vi "CAL-Interp.vi"(0 "Frequency (Hz)":dbl[](array[numeric]), 5 "Magnitude (dB)":dbl[](array[numeric]), 7 "Phase (degrees)":dbl[](array[numeric]), 9 "df (Hz)":dbl) -> (4 "Interp Freq (Hz)":dbl[](array[numeric]), 6 "Interp Magnitude (dB)":dbl[](array[numeric]), 8 "Interp Phase (degrees)":dbl[](array[numeric]), 15 "Interp z":cdb[](array[numeric]))   [LabVIEW 2020]
uses:
  epl-vi-lib/Utility VIs/Math VIs/dB to Linear (1D).vi
  epl-vi-lib/Utility VIs/Math VIs/LinSpace (start-stop-step).vi
  epl-vi-lib/Utility VIs/Math VIs/Linear to dB (array).vi
  <vilib>/gmath/NI_Gmath.lvlib
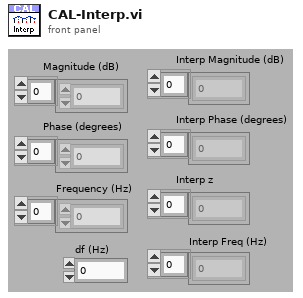
[diagram p1: front panel]
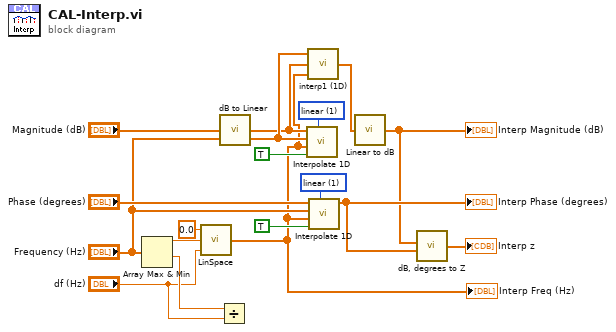
[diagram p0: block diagram]
diagram:
  w13 = 1 items=["nearest", "linear", "spline", "cubic Hermite", "Lagrange"] ("method")
  w17 = 1 items=["nearest", "linear", "spline", "cubic Hermite", "Lagrange"] ("method")
  n1 = Array Max & Min(array="Frequency (Hz)") -> (max value=w15:dbl, min value=w6:dbl)  [unwired: 2 out]
  n2 = call-poly "LinSpace.vi"("Step"="df (Hz)", "Stop"=w15, "Start"=0.0) -> ("Array"=w2:dbl[])  [unwired: 1 in, 1 out]
  "Interp Freq (Hz)" <- w2
  n3 = Divide(x=w6, y="df (Hz)") -> ()  [unwired: 1 out]
  n4 = call-poly "dB to Linear.vi"("dB"="Magnitude (dB)") -> ("linear"=w3:dbl[])
  n5 = call <vilib>:"Interpolate 1D.vi"("method"=w17, "X is monotonic"=TRUE, "xi"=w2, "X"="Frequency (Hz)", "Y"=w3) -> ()  [unwired: 4 in, 3 out]
  n6 = call "interp1 (1D).vi"("X"="Frequency (Hz)", "Y"=w3, "U"=w2) -> ("V"=w1:dbl[])  [unwired: 2 in]
  n7 = call <vilib>:"Interpolate 1D.vi"("method"=w13, "X is monotonic"=TRUE, "xi"=w2, "X"="Frequency (Hz)", "Y"="Phase (degrees)") -> ("yi"=w10:dbl[])  [unwired: 4 in, 2 out]
  "Interp Phase (degrees)" <- w10
  n8 = call-poly "Linear to dB.vi"("linear"=w1) -> ("dB"=w8:dbl[])
  "Interp Magnitude (dB)" <- w8
  n9 = call "dB, degrees to Z.vi"("Magnitude (dB)"=w8, "Phase (degrees)"=w10) -> ("Z"=→"Interp z":cdb[])  [unwired: 5 in]
